vi "Begin.vi"(11 "Image Size":T1=enum."160x120") -> (0 "error out":errorcluster)   [LabVIEW 2011]
doc: "Called before other user functions, this VI is expected to open initial I/O refnums, load in file data, and do all program initialization. Notice that the <B>error out</B> terminal is simply used for data flow. Wiring it to other structures or subVIs ensures that this VI runs first."
uses:
  <vilib>/Rock Robotics/WPI/Camera/WPI_CameraImageSize.ctl
  <vilib>/Rock Robotics/SystemInterfaces/DIO/FPGA_DIOPWMChannel.ctl
  <vilib>/Rock Robotics/WPI/Joystick/WPI_JoystickDeviceEnum.ctl
  <vilib>/Rock Robotics/WPI/Camera/WPI_CameraWhite Balance Values.ctl
  <vilib>/Rock Robotics/WPI/Camera/WPI_CameraExposure Values.ctl
  <vilib>/Rock Robotics/WPI/Camera/WPI_CameraFrameRate.ctl
  <vilib>/Rock Robotics/SystemInterfaces/DIO/FPGA_DIOChannel.ctl
  <vilib>/Rock Robotics/SystemInterfaces/Typedef/FPGA_TypedefDigitalModule.ctl
  <vilib>/Rock Robotics/WPI/RobotDrive/WPI_RobotDriveOpen2MotorWithJaguar.vi
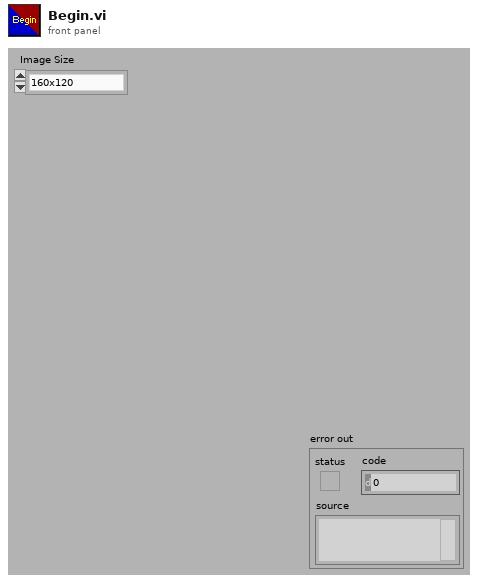
[diagram p1: front panel]
types:
  T1 = typedef "WPI_CameraImageSize.ctl" = enum16{"640x480", "320x240", "160x120"}
  T2 = typedef "FPGA_TypedefDigitalModule.ctl" = enum16{"Digital Module 1", "Digital Module 2"}
  T3 = typedef "FPGA_DIOChannel.ctl" = enum8{"DIO 1", "DIO 2", "DIO 3", "DIO 4", "DIO 5", "DIO 6", "DIO 7", "DIO 8", "DIO 9", "DIO 10", "DIO 11", "DIO 12", "DIO 13", "DIO 14", "Invalid"}
  T4 = typedef "WPI_CameraFrameRate.ctl" = u32
  T5 = typedef "WPI_CameraExposure Values.ctl" = enum16{"Auto", "Flicker-free 50 Hz", "Flicker-free 60 Hz", "Hold current"}
  T6 = typedef "WPI_CameraWhite Balance Values.ctl" = enum16{"Auto", "Fixed indoor", "Fixed outdoor 1", "Fixed outdoor 2", "Fixed fluorescent 1", "Fixed fluorescent 2", "Hold current"}
  T7 = typedef "WPI_JoystickDeviceEnum.ctl" = enum16{"USB 1", "USB 2", "USB 3", "USB 4", "Kinect 1", "Kinect 2"}
  T8 = typedef "FPGA_DIOPWMChannel.ctl" = enum8{"PWM 1", "PWM 2", "PWM 3", "PWM 4", "PWM 5", "PWM 6", "PWM 7", "PWM 8", "PWM 9", "PWM 10", "Invalid"}
  T9 = typedef "WPI_CameraDevRef.ctl" = cluster{"Camera Address":string, "CameraStatus":errorcluster, "Acquire Image Notifier":refnum<notifier>}
  T10 = typedef "WPI_RobotDriveDevRef.ctl" = cluster{"DevStatus":errorcluster, "Motors[]":T11[], "Square Inputs":bool, "Max Output":dbl, "Isochronous":bool}
  T11 = typedef "WPI_MotorControlDeviceRef.ctl" = cluster{"DeviceStatus":errorcluster, "Type":enum16{"PWM", "CAN"}, "PWM":cluster{"Digital Module":T2, "PWM Channel":T8, "DeadBand":T12}, "CAN":cluster{"Device Number":u8, "Control Mode":T13, "Semaphore":T14, "Max Vout":dbl}, "Invert":bool, "TransformRef":T15, "InvTransformRef":T15}
  T12 = typedef "WPI_PWMDeadband.ctl" = cluster{"Name":string, "maxPositivePwm":i32, "minPositivePwm":i32, "centerPwm":i32, "maxNegativePwm":i32, "minNegativePwm":i32, "angularRange":u16}
  T13 = typedef "WPI_CANJaguar_ControlMode.ctl" = enum8{"Percent VBus", "Current", "Speed", "Position", "Voltage"}
  T14 = typedef "Semaphore RefNum" = refnum<k1>
  T15 = typedef "WPI_PWMTransform_ConPane.ctl" = refnum<vi>
  T16 = typedef "WPI_JoystickDevRef.ctl" = cluster{"Device":T7}
  T17 = typedef "WPI_DigitalInputDevRef.ctl" = cluster{"DevStatus":errorcluster, "DIO Channel":T3, "Digital Module":T2}
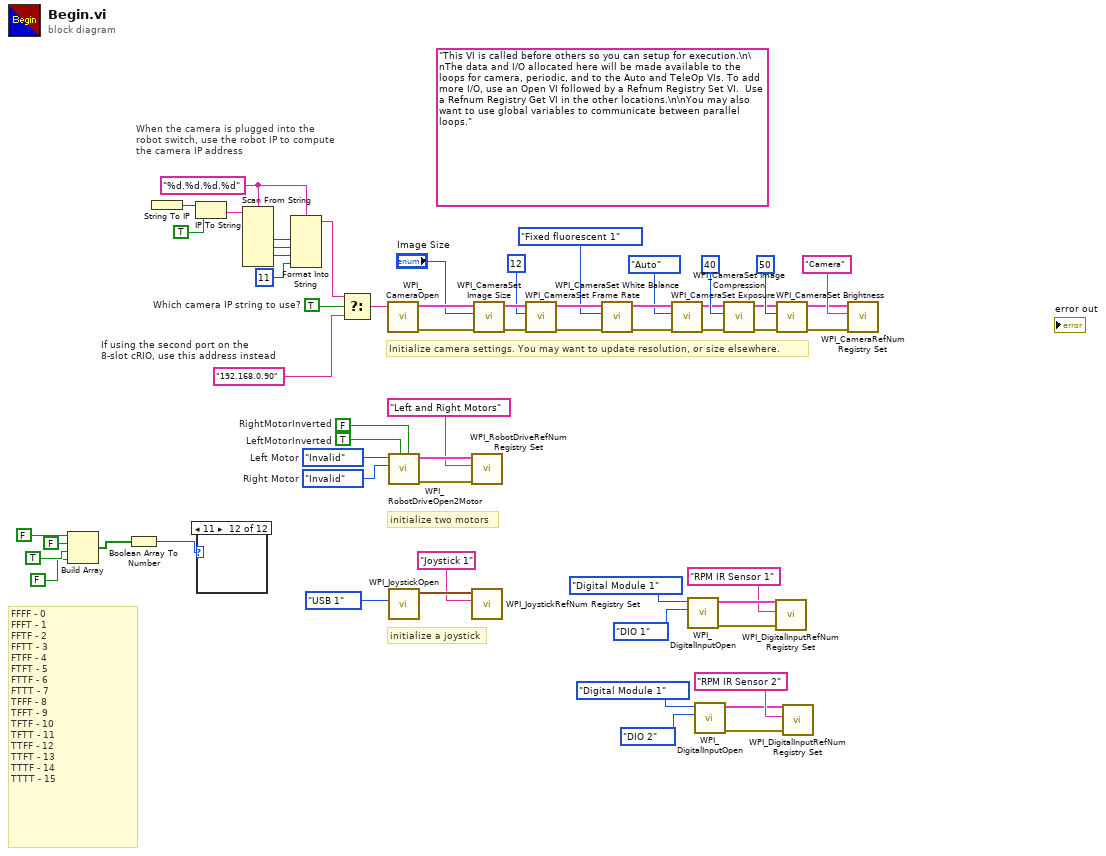
[diagram p0: block diagram]
diagram:
  w17 = TRUE  # Which camera IP string to use?
  w21 = "%d.%d.%d.%d" ("format string")
  (unwired) "This VI is called before others so you can setup for execution.\n\nThe data and I/O allocated here will be made available to the loops for camera, periodic, and to the Auto and TeleOp VIs. To add more I/O, use an Open VI followed by a Refnum Registry Set VI.  Use a Refnum Registry Get VI in the other locations.\n\nYou may also want to use global variables to communicate between parallel loops."
  w33 = FPGA_DIOPWMChannel."Invalid"  # Right Motor
  w34 = FPGA_DIOPWMChannel."Invalid"  # Left Motor
  w18 = "192.168.0.90"  # If using the second port on the 8-slot cRIO, use this address instead
  w58 = TRUE  # LeftMotorInverted
  w59 = FALSE  # RightMotorInverted
  # "FFFF - 0\nFFFT - 1\nFFTF - 2\nFFTT - 3\nFTFF - 4\nFTFT - 5\nFTTF - 6\nFTTT - 7\nTFFF - 8\nTFFT - 9\nTFTF - 10\nTFTT - 11\nTTFF - 12\nTTFT - 13\nTTTF - 14\nTTTT - 15"
  # "When the camera is plugged into the\nrobot switch, use the robot IP to compute\nthe camera IP address"
  # "initialize a joystick"
  # "initialize two motors"
  # "Initialize camera settings. You may want to update resolution, or size elsewhere."
  n1 = Build Array(FALSE, FALSE ("element"), TRUE ("element"), FALSE ("element")) -> (w2:bool[])
  n2 = Boolean Array To Number(Boolean array=w2) -> (number=w1:u32)
  n3 = String To IP() -> (0:w28:u32)  [unwired: 1 in]
  n4 = IP To String(1:TRUE ("dot notation? (F)"), 2:w28) -> (0:w26:string)
  n5 = case shown="11" w1 {
    frame 0, Default {
    }
    frame 1 {
    }
    frame 2 {
    }
    frame 3 {
    }
    frame 4 {
    }
    frame 5 {
    }
    frame 6 {
    }
    frame 7 {
    }
    frame 8 {
    }
    frame 9 {
    }
    frame 10 {
    }
    frame 11 {
    }
  }
  n6 = Scan From String(format string=w21, input string=w26) -> (output 1=w25:i32, output 2=w24:i32, output 3=w23:i32)  [unwired: 7 in, 3 out]
  n7 = Format Into String(format string=w21, w25, w24, w23, 11 ("Compression")) -> (resulting string=w19:string)  [unwired: 2 in, 1 out]
  n8 = Select(t=w19, s=w17, f=w18) -> (s? t:f=w20:string)
  n9 = call <vilib>:"WPI_CameraOpen.vi"("Camera Address"=w20) -> ("error out"=w43:errorcluster, "CameraDevRef"=w44:T9)  [unwired: 1 in, 8 out]
  n10 = call-poly <vilib>:"WPI_RobotDriveOpen2Motor.vi"("Right Motor Inverted"=w59, "Left Motor Inverted"=w58, "Right Motor"=w33, "Left Motor"=w34) -> ("error out"=w52:errorcluster, "RobotDriveDevRef"=w56:T10)  [unwired: 1 in, 5 out]
  n11 = call <vilib>:"WPI_JoystickOpen.vi"("JoystickDevice"=WPI_JoystickDeviceEnum."USB 1") -> ("JoystickDevRef"=w54:T16)  [unwired: 10 out]
  n12 = call <vilib>:"WPI_RobotDriveRefNum Registry Set.vi"("error in (no error)"=w52, "refnum name"="Left and Right Motors", "RobotDriveDevRef"=w56) -> ()  [unwired: 9 out]
  n13 = call <vilib>:"WPI_JoystickRefNum Registry Set.vi"("refnum name"="Joystick 1", "JoystickDevRef"=w54) -> ()  [unwired: 1 in, 9 out]
  n14 = call <vilib>:"WPI_CameraSet Image Size.vi"("error in (no error)"=w43, "Image Size"="Image Size", "CameraDevRef"=w44) -> ("error out"=w42:errorcluster, "CameraDevRef Out"=w45:T9)  [unwired: 7 out]
  n15 = call <vilib>:"WPI_CameraSet Frame Rate.vi"("error in (no error)"=w42, "Frame Rate (fps)"=T4 12, "CameraDevRef"=w45) -> ("error out"=w41:errorcluster, "CameraDevRef Out"=w47:T9)  [unwired: 7 out]
  n16 = call <vilib>:"WPI_CameraSet White Balance.vi"("error in (no error)"=w41, "White Balance"=WPI_CameraWhite_Balance_Values."Fixed fluorescent 1", "CameraDevRef"=w47) -> ("error out"=w40:errorcluster, "CameraDevRef Out"=w46:T9)  [unwired: 7 out]
  n17 = call <vilib>:"WPI_CameraSet Exposure.vi"("error in (no error)"=w40, "Exposure"=WPI_CameraExposure_Values."Auto", "CameraDevRef"=w46) -> ("error out"=w39:errorcluster, "CameraDevRef Out"=w49:T9)  [unwired: 7 out]
  n18 = call <vilib>:"WPI_DigitalInputOpen.vi"("DIO Channel"=FPGA_DIOChannel."DIO 1", "Digital Module (Module 1)"=FPGA_TypedefDigitalModule."Digital Module 1") -> ("error out"=w13:errorcluster, "DigitalInputDevRef"=w14:T17)  [unwired: 8 in]
  n19 = call <vilib>:"WPI_DigitalInputOpen.vi"("DIO Channel"=FPGA_DIOChannel."DIO 2", "Digital Module (Module 1)"=FPGA_TypedefDigitalModule."Digital Module 1") -> ("error out"=w10:errorcluster, "DigitalInputDevRef"=w9:T17)  [unwired: 8 in]
  n20 = call <vilib>:"WPI_CameraSet Image Compression.vi"("error in (no error)"=w39, "Compression"=40, "CameraDevRef"=w49) -> ("error out"=w38:errorcluster, "CameraDevRef Out"=w48:T9)  [unwired: 7 out]
  n21 = call <vilib>:"WPI_DigitalInputRefNum Registry Set.vi"("error in (no error)"=w13, "refnum name"="RPM IR Sensor 1", "DigitalInputDevRef"=w14) -> ()  [unwired: 7 in, 2 out]
  n22 = call <vilib>:"WPI_CameraSet Brightness.vi"("error in (no error)"=w38, "Brightness"=50, "CameraDevRef"=w48) -> ("error out"=w36:errorcluster, "CameraDevRef Out"=w37:T9)  [unwired: 7 out]
  n23 = call <vilib>:"WPI_DigitalInputRefNum Registry Set.vi"("error in (no error)"=w10, "refnum name"="RPM IR Sensor 2", "DigitalInputDevRef"=w9) -> ()  [unwired: 7 in, 2 out]
  n24 = call <vilib>:"WPI_CameraRefNum Registry Set.vi"("error in (no error)"=w36, "refnum name"="Camera", "CameraDevRef"=w37) -> ()  [unwired: 9 out]
